vi "ALTS-2015 Authentication Screen.vi"(8 "error in (no error)":errorcluster) -> (0 "error IO":errorcluster, 1 "User Group":T1, 2 "User Name":string, 3 "Valid Login?":bool)   [LabVIEW 2013]
uses:
  Controls/ALTS User Group Enum2.ctl
  Controls/ALTS Poll Control Autentication.ctl
panel:
  out "Time":string
  out "User Group":T1
  in  "Delete":bool
  in  "Edit":bool
  in  "Add":bool
  in  "Cancel":bool
  in  "OK":bool
  in  "Password":string
  in  "User Name":i32(ring) items=["Administrator", "oper", "Ajayvignesh"]
  # "Authentication Screen"
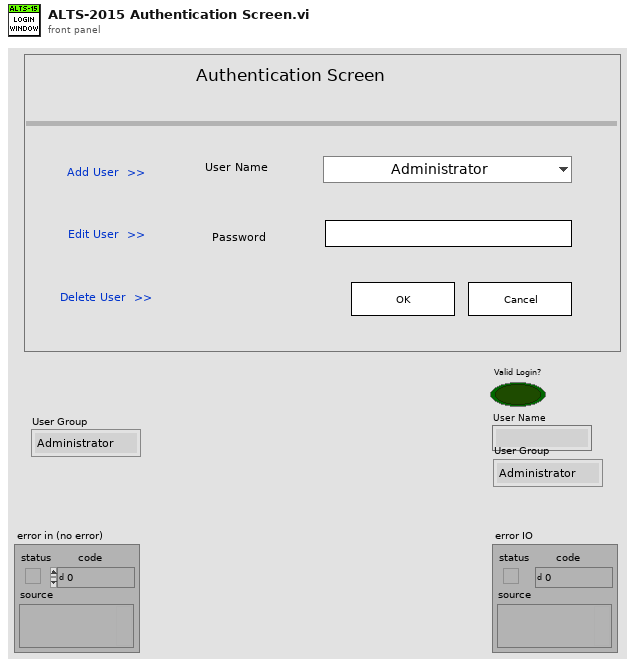
[diagram p1: front panel]
types:
  T1 = typedef "ALTS User Group Enum2.ctl" = enum16{"Administrator", "Super User", "Operator"}
  T2 = typedef "ALTS Poll Control Autentication.ctl" = enum16{">Initialize", ">ReInitialize", ">Poll", ">Handle Error", ">User Name Changed", ">Verify Password", ">On OK", ">On Cancel", ">Add User", ">Edit User", ">Delete User", ">Close Handle", ">NOP", ">Exit"}
  T3 = cluster{"User Names":string, "Password":string, "User Rights":T1}[]
  T4 = typedef "eventvkey.ctl" = enum16{"ASCII", "Enter", "Return", "Shift", "Ctrl", "Alt", "Cmd", "Opt", "Caps", "NumLock", "Clear", "Break", "Up", "Down", "Left", "Right", "Insert", "Delete", "Home", "End", "PageUp", "PageDown", "Escape", "Help", "Pause", "ScrollLock", "F1", "F2", "F3", "F4", "F5", "F6", "F7", "F8", "F9", "F10", "F11", "F12", "F13", "F14", "F15", "F16", "F17", "F18", "F19", "F20", "F21", "F22", "F23", "F24", "Play", "VolumeUp", "VolumeDown", "Mute", "Two Byte Char"}
  T5 = enum16{"OK", "CANCEL", "ABORT", "RETRY", "IGNORE", "YES", "NO"}
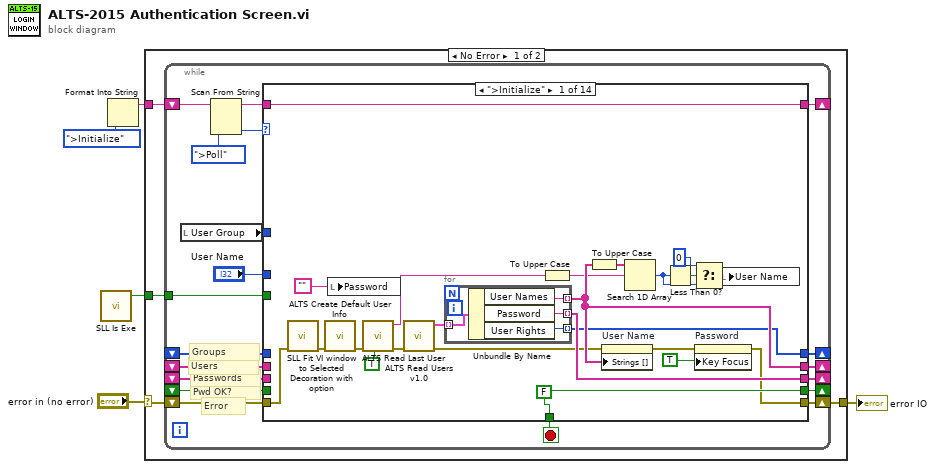
[diagram p0: block diagram]
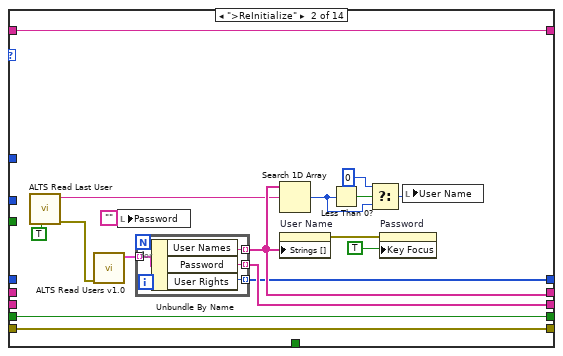
[diagram p2: hidden frame]
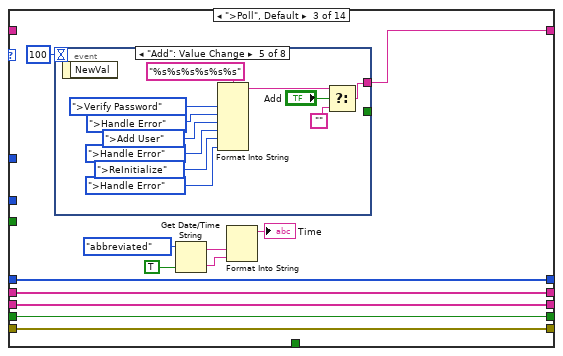
[diagram p3: hidden frame]
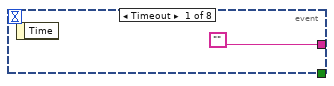
[diagram p4: hidden frame]
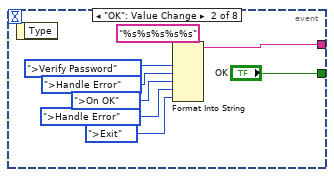
[diagram p5: hidden frame]
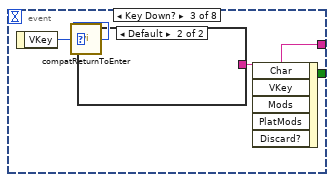
[diagram p6: hidden frame]
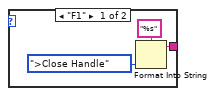
[diagram p7: hidden frame]
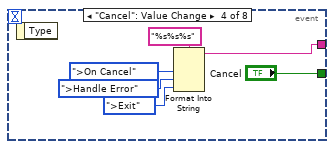
[diagram p8: hidden frame]
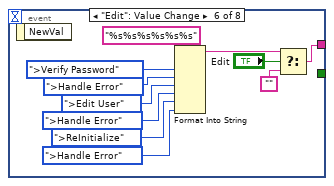
[diagram p9: hidden frame]
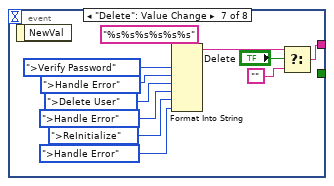
[diagram p10: hidden frame]
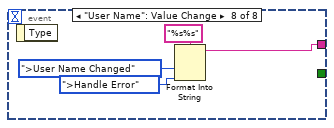
[diagram p11: hidden frame]
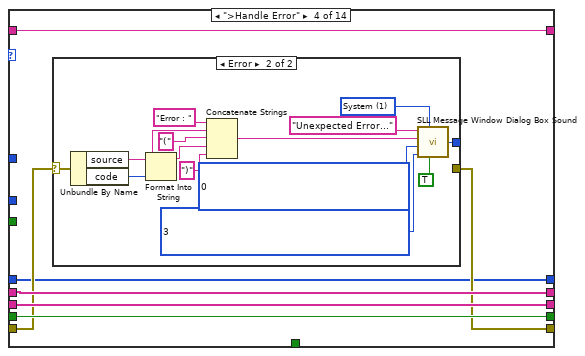
[diagram p12: hidden frame]
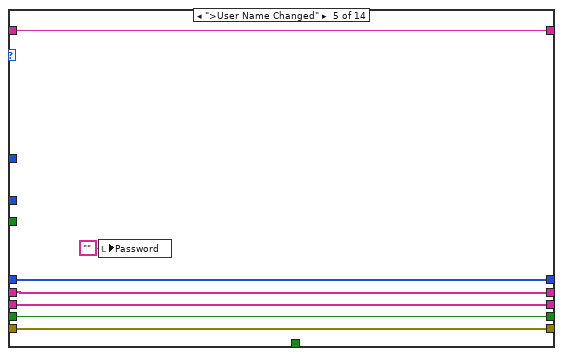
[diagram p14: hidden frame]
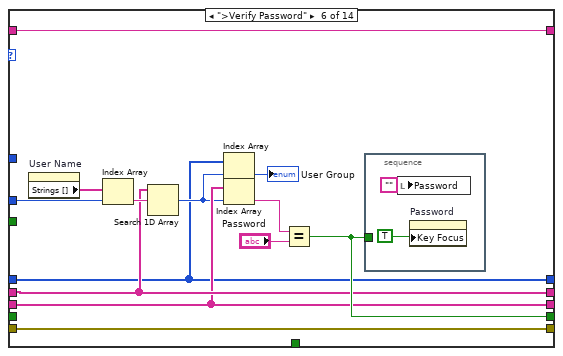
[diagram p15: hidden frame]
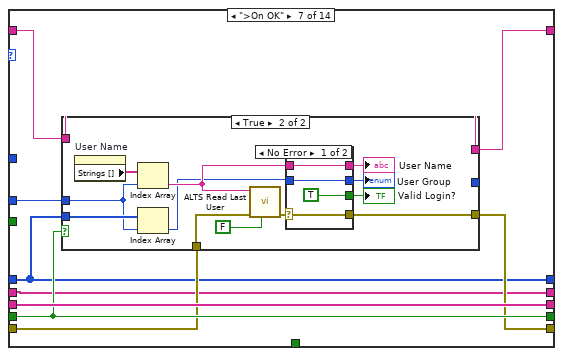
[diagram p16: hidden frame]
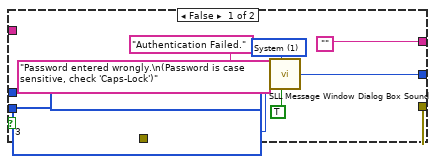
[diagram p17: hidden frame]
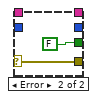
[diagram p18: hidden frame]
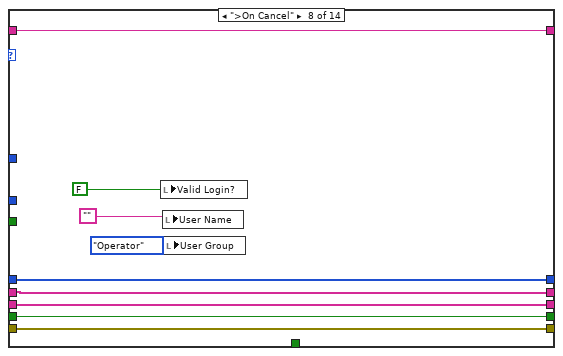
[diagram p19: hidden frame]
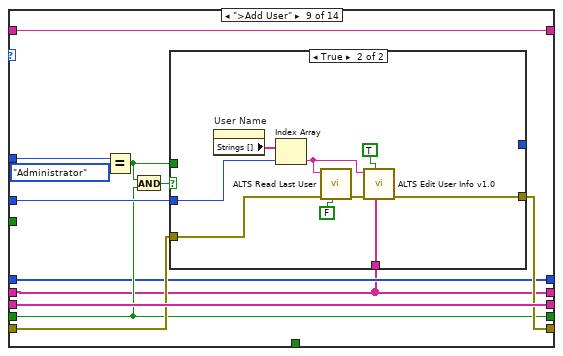
[diagram p20: hidden frame]
diagram:
  n1 = call <userlib>:"SLL Is Exe.vi"() -> ("Is Exe?"=w1:bool)  [unwired: 10 in, 1 out]
  n2 = Format Into String(ALTS_Poll_Control_Autentication.">Initialize" ("Poll Enum Autenticatin")) -> (resulting string=w2:string)  [unwired: 3 in, 1 out]
  n3 = case shown="No Error" "error in (no error)" {
    selector: "error in (no error)" -> [w9 w353]
    tunnel: [w8 w353] -> w4
    tunnel: w2 -> [w7 _]
    tunnel: w1 -> [w6 _]
    frame No Error {
      n4 = while {
        shift-right: [w27] -> w8
        shift-left: w9 -> [w28]
        shift-right: [w22] -> _
        shift-left: w7 -> [w25]
        shift-right: [w16] -> _
        shift-left: _ -> [w15]
        shift-right: [w17] -> _
        shift-left: _ -> [w18]
        shift-right: [w19] -> _
        shift-left: _ -> [w20]
        tunnel: w6 -> [w14]
        shift-right: [w10] -> _
        shift-left: _ -> [w11]
        stop <- w21 stop-if-true
        # "Error"
        # "Pwd OK?"
        # "Passwords"
        # "Users"
        # "Groups"
        n5 = local read "User Group"() -> (w13:T1)
        n6 = Scan From String(input string=w25, default 1=ALTS_Poll_Control_Autentication.">Poll" ("Poll Enum Autenticatin")) -> (remaining string=w23:string, output 1=w24:T2)  [unwired: 3 in, 2 out]
        n7 = case shown="\">Initialize\"" w24 {
          tunnel: [w46 w71 w77 w148 w174 w183 w196 w233 w245 w275 w302 w334 w344 w347] -> w27
          tunnel: w28 -> [w29 w71 w77 w149 w174 w183 w197 w233 w246 w276 w303 w334 w344 w347]
          tunnel: w23 -> [w51 w72 _ w153 w175 w188 w194 w231 w248 w279 w307 w339 w345 w352]
          tunnel: [w51 w72 w78 w153 w175 w188 w193 w231 w248 w279 w307 w339 w345 w352] -> w22
          tunnel: [w49 _ _ _ _ _ _ _ _ _ _ _ _ TRUE] -> w21
          tunnel: w20 -> [_ _ w88 w150 w171 w182 w191 w234 w237 w271 w305 w336 w341 w349]
          tunnel: [w50 w70 w88 w150 w171 w182 w191 w234 w237 w271 w305 w336 w341 w349] -> w19
          tunnel: w18 -> [_ _ w84 w151 w172 w181 w199 w235 w247 w278 w306 w337 w342 w350]
          tunnel: [w48 w69 w84 w151 w172 w181 w199 w235 w247 w278 w306 w337 w342 w350] -> w17
          tunnel: [w49 w67 w87 w152 w173 w185 w198 w236 w242 w277 w304 w338 w343 w351] -> w16
          tunnel: w15 -> [_ w67 w87 w152 w173 _ w198 w236 w242 w277 w304 w338 w343 w351]
          tunnel: w14 -> [_ _ _ _ _ _ _ _ _ _ _ _ _ _]
          tunnel: "User Name" -> [_ _ _ _ _ w184 w195 _ w244 w274 w301 _ _ _]
          tunnel: w13 -> [_ _ _ _ _ _ _ _ w241 w273 w299 _ _ _]
          tunnel: w11 -> [_ _ w85 w147 w169 w179 w192 w232 w238 w272 w300 w335 w340 w348]
          tunnel: [w47 w68 w85 w147 w169 w179 w192 w232 w238 w272 w300 w335 w340 w348] -> w10
          frame ">Initialize" {
            w49 = FALSE
            n8 = call <userlib>:"SLL Fit VI window to Selected Decoration with option.vi"("error in (no error)"=w29) -> ("error out"=w30:errorcluster)  [unwired: 9 in, 1 out]
            n9 = call "ALTS Create Default User Info.vi"("error in"=w30) -> ("error out"=w31:errorcluster)  [unwired: 10 in]
            n10 = local write "Password"("" ("Password")) -> ()
            n11 = call "ALTS Read Last User.vi"("Read?"=TRUE, "error in (no error)"=w31) -> ("error out"=w37:errorcluster, "Last User"=w38:string)  [unwired: 8 in]
            n12 = call "ALTS Read Users v1.0.vi"("error in (no error)"=w37) -> ("error out"=w39:errorcluster, "Users"=w40:T3)  [unwired: 9 in]
            n13 = for {
              tunnel: w40 -> [w55] mode=indexing
              tunnel: [w54] -> w50 mode=indexing
              tunnel: [w53] -> w48 mode=indexing
              tunnel: [w52] -> w47 mode=indexing
              n14 = Unbundle By Name(w55) -> ("User Names"=w54:string, "Password"=w53:string, "User Rights"=w52:T1)
            }
            n15 = To Upper Case(1:w38) -> (0:w41:string)
            n16 = To Upper Case(1:w50) -> (0:w42:string[])
            n17 = property on="User Name" class="Ring (strict)"(error in=w39, "Strings []"=w50) -> (error out=w44:errorcluster)  [unwired: 1 in, 1 out]
            n18 = Search 1D Array(1D array=w42, element=w41) -> (index of element=w33:i32)  [unwired: 1 in]
            n19 = Less Than 0?(x=w33) -> (x < 0?=w35:bool)
            n20 = Select(t=0, s=w35, f=w33) -> (s? t:f=w34:i32)
            n21 = property on="Password" class="Str"(error in=w44, "Key Focus"=TRUE) -> (error out=w46:errorcluster)  [unwired: 1 in, 1 out]
            n22 = local write "User Name"(w34) -> ()
          }
          frame ">ReInitialize" {
            n23 = call "ALTS Read Last User.vi"("Read?"=TRUE) -> ("error out"=w61:errorcluster, "Last User"=w62:string)  [unwired: 9 in]
            n24 = call "ALTS Read Users v1.0.vi"("error in (no error)"=w61) -> ("Users"=w63:T3)  [unwired: 9 in, 1 out]
            n25 = local write "Password"("" ("Password")) -> ()
            n26 = for {
              tunnel: w63 -> [w76] mode=indexing
              tunnel: [w75] -> w70 mode=indexing
              tunnel: [w74] -> w69 mode=indexing
              tunnel: [w73] -> w68 mode=indexing
              n27 = Unbundle By Name(w76) -> ("User Names"=w75:string, "Password"=w74:string, "User Rights"=w73:T1)
            }
            n28 = Search 1D Array(1D array=w70, element=w62) -> (index of element=w58:i32)  [unwired: 1 in]
            n29 = property on="User Name" class="Ring (strict)"("Strings []"=w70) -> (error out=w65:errorcluster)  [unwired: 2 in, 1 out]
            n30 = Less Than 0?(x=w58) -> (x < 0?=w59:bool)
            n31 = Select(t=0, s=w59, f=w58) -> (s? t:f=w56:i32)
            n32 = property on="Password" class="Str"(error in=w65, "Key Focus"=TRUE) -> ()  [unwired: 1 in, 2 out]
            n33 = local write "User Name"(w56) -> ()
          }
          frame ">Poll", Default {
            n34 = event shown="[4] \"Add\": Value Change" {
              selector: _ -> [_ _ _ _ _ _ _ _]
              dyn-events: _ -> [_ _ _ _ _ _ _ _]
              timeout: 100 -> [_ _ _ _ _ _ _ _]
              tunnel: [_ "OK" _ "Cancel" _ _ _ _] -> _
              tunnel: ["" w94 w99 w107 w111 w122 w133 w144] -> w78
              event Timeout {
                n35 = event-data() -> ()  [unwired: 1 in, 1 out]
              }
              event "OK": Value Change {
                n36 = event-data() -> ()  [unwired: 1 in, 1 out]
                n37 = Format Into String(format string="%s%s%s%s%s", ALTS_Poll_Control_Autentication.">Verify Password" ("Poll Enum Autenticatin"), ALTS_Poll_Control_Autentication.">Handle Error" ("Poll Enum Autenticatin"), ALTS_Poll_Control_Autentication.">On OK" ("Poll Enum Autenticatin"), ALTS_Poll_Control_Autentication.">Handle Error" ("Poll Enum Autenticatin"), ALTS_Poll_Control_Autentication.">Exit" ("Poll Enum Autenticatin")) -> (resulting string=w94:string)  [unwired: 2 in, 1 out]
              }
              event Key Down? {
                n38 = event-data() -> ("VKey"=w98:T4)  [unwired: 1 in]
                n39 = call <vilib>:"compatReturnToEnter.vi"("VKey"=w98) -> ("VKey"=w100:T4)
                n40 = case shown="Default" w100 {
                  tunnel: [w101 _] -> w99
                  frame "F1" {
                    n41 = Format Into String(format string="%s", ALTS_Poll_Control_Autentication.">Close Handle" ("Poll Enum Autenticatin")) -> (resulting string=w101:string)  [unwired: 2 in, 1 out]
                  }
                  frame Default {
                  }
                }
                n42 = event-data() -> ()  [unwired: 6 in, 1 out]
              }
              event "Cancel": Value Change {
                n43 = event-data() -> ()  [unwired: 1 in, 1 out]
                n44 = Format Into String(format string="%s%s%s", ALTS_Poll_Control_Autentication.">On Cancel" ("Poll Enum Autenticatin"), ALTS_Poll_Control_Autentication.">Handle Error" ("Poll Enum Autenticatin"), ALTS_Poll_Control_Autentication.">Exit" ("Poll Enum Autenticatin")) -> (resulting string=w107:string)  [unwired: 2 in, 1 out]
              }
              event "Add": Value Change {
                n45 = event-data() -> ()  [unwired: 1 in, 1 out]
                n46 = Format Into String(format string="%s%s%s%s%s%s", ALTS_Poll_Control_Autentication.">Verify Password" ("Poll Enum Autenticatin"), ALTS_Poll_Control_Autentication.">Handle Error" ("Poll Enum Autenticatin"), ALTS_Poll_Control_Autentication.">Add User" ("Poll Enum Autenticatin"), ALTS_Poll_Control_Autentication.">Handle Error" ("Poll Enum Autenticatin"), ALTS_Poll_Control_Autentication.">ReInitialize" ("Poll Enum Autenticatin"), ALTS_Poll_Control_Autentication.">Handle Error" ("Poll Enum Autenticatin")) -> (resulting string=w113:string)  [unwired: 2 in, 1 out]
                n47 = Select(t=w113, s="Add", f="") -> (s? t:f=w111:string)
              }
              event "Edit": Value Change {
                n48 = event-data() -> ()  [unwired: 1 in, 1 out]
                n49 = Format Into String(format string="%s%s%s%s%s%s", ALTS_Poll_Control_Autentication.">Verify Password" ("Poll Enum Autenticatin"), ALTS_Poll_Control_Autentication.">Handle Error" ("Poll Enum Autenticatin"), ALTS_Poll_Control_Autentication.">Edit User" ("Poll Enum Autenticatin"), ALTS_Poll_Control_Autentication.">Handle Error" ("Poll Enum Autenticatin"), ALTS_Poll_Control_Autentication.">ReInitialize" ("Poll Enum Autenticatin"), ALTS_Poll_Control_Autentication.">Handle Error" ("Poll Enum Autenticatin")) -> (resulting string=w124:string)  [unwired: 2 in, 1 out]
                n50 = Select(t=w124, s="Edit", f="") -> (s? t:f=w122:string)
              }
              event "Delete": Value Change {
                n51 = event-data() -> ()  [unwired: 1 in, 1 out]
                n52 = Format Into String(format string="%s%s%s%s%s%s", ALTS_Poll_Control_Autentication.">Verify Password" ("Poll Enum Autenticatin"), ALTS_Poll_Control_Autentication.">Handle Error" ("Poll Enum Autenticatin"), ALTS_Poll_Control_Autentication.">Delete User" ("Poll Enum Autenticatin"), ALTS_Poll_Control_Autentication.">Handle Error" ("Poll Enum Autenticatin"), ALTS_Poll_Control_Autentication.">ReInitialize" ("Poll Enum Autenticatin"), ALTS_Poll_Control_Autentication.">Handle Error" ("Poll Enum Autenticatin")) -> (resulting string=w135:string)  [unwired: 2 in, 1 out]
                n53 = Select(t=w135, s="Delete", f="") -> (s? t:f=w133:string)
              }
              event "User Name": Value Change {
                n54 = event-data() -> ()  [unwired: 1 in, 1 out]
                n55 = Format Into String(format string="%s%s", ALTS_Poll_Control_Autentication.">User Name Changed" ("Poll Enum Autenticatin"), ALTS_Poll_Control_Autentication.">Handle Error" ("Poll Enum Autenticatin")) -> (resulting string=w144:string)  [unwired: 2 in, 1 out]
              }
            }
            n56 = Get Date/Time String(date format (0)=enum16{"short", "long", "abbreviated"}."abbreviated", want seconds? (F)=TRUE) -> (date string=w82:string, time string=w81:string)  [unwired: 1 in]
            n57 = Format Into String(w82, w81) -> (resulting string=→"Time":string)  [unwired: 3 in, 1 out]
          }
          frame ">Handle Error" {
            n58 = case shown="Error" w149 {
              selector: w149 -> [w154 w163]
              tunnel: [w154 _] -> w148
              tunnel: [_ w155] -> _
              frame No Error {
              }
              frame Error {
                w165 = 1 items=["Application", "System", "Task"] ("modality (0)")
                n59 = Unbundle By Name(w163) -> ("source"=w161:string, "code"=w162:i32)
                n60 = Format Into String(w162) -> (resulting string=w160:string)  [unwired: 3 in, 1 out]
                n61 = Concatenate Strings("Error : " ("string"), w161, "(" ("string"), w160, ")" ("string")) -> (w156:string)
                n62 = call <userlib>:"SLL Message Window Dialog Box Sound.vi"("Sound? (F)"=TRUE ("sound? (F)"), "Modality (0)"=w165, "Icon (0:None)"=3 ("icon (0:None)"), "Buttons (0:OK)"=0 ("buttons (0:OK)"), "Message (\"\")"=w156, "Window Title (\"\")"="Unexpected Error..." ("window title (\"\")")) -> ("Button Pressed"=w155:T5)
              }
            }
          }
          frame ">User Name Changed" {
            n63 = local write "Password"("") -> ()
          }
          frame ">Verify Password" {
            n64 = property on="User Name" class="Ring (strict)"() -> ("Strings []"=w186:string[])  [unwired: 2 in, 2 out]
            n65 = Index Array(array=w186, index=w184) -> (element=w187:string)
            n66 = Search 1D Array(1D array=w182, element=w187) -> (index of element=w180:i32)  [unwired: 1 in]
            n67 = Index Array(array=w179, index=w180) -> (element=→"User Group":T1)
            n68 = Index Array(array=w181, index=w180) -> (element=w177:string)
            n69 = Equal?(x=w177, y="Password") -> (x = y?=w185:bool)
            n70 = stacked-sequence {
              tunnel: w185 -> [_]
              frame #0 {
                n71 = local write "Password"("" ("Password")) -> ()
                n72 = property on="Password" class="Str"("Key Focus"=TRUE) -> ()  [unwired: 2 in, 2 out]
              }
            }
          }
          frame ">On OK" {
            n73 = case shown="True" w198 {
              tunnel: [w208 _] -> _
              tunnel: w197 -> [w201 w219]
              tunnel: [w201 w213] -> w196
              tunnel: w195 -> [_ w214]
              tunnel: ["" w218] -> w193
              tunnel: w194 -> [_ w218]
              tunnel: w192 -> [_ w216]
              frame False {
                w203 = 1 items=["Application", "System", "Task"] ("modality (0)")
                n74 = call <userlib>:"SLL Message Window Dialog Box Sound.vi"("Sound? (F)"=TRUE ("sound? (F)"), "Modality (0)"=w203, "Icon (0:None)"=3 ("icon (0:None)"), "Buttons (0:OK)"=0 ("buttons (0:OK)"), "Message (\"\")"="Password entered wrongly.\n(Password is case sensitive, check 'Caps-Lock')" ("message (\"\")"), "Window Title (\"\")"="Authentication Failed." ("window title (\"\")")) -> ("Button Pressed"=w208:T5)
              }
              frame True {
                n75 = property on="User Name" class="Ring (strict)"() -> ("Strings []"=w221:string[])  [unwired: 2 in, 2 out]
                n76 = Index Array(array=w221, index=w214) -> (element=w217:string)
                n77 = Index Array(array=w216, index=w214) -> (element=w210:T1)
                n78 = call "ALTS Read Last User.vi"("Read?"=FALSE, "error in (no error)"=w219, "Last User"=w217) -> ("error out"=w215:errorcluster)  [unwired: 7 in, 1 out]
                n79 = case shown="No Error" w215 {
                  selector: w215 -> [w225 w226]
                  tunnel: w217 -> [w223 _]
                  tunnel: w210 -> [w222 _]
                  tunnel: [w225 w226] -> w213
                  tunnel: [TRUE ("Valid Login?") FALSE ("Valid Login?")] -> w209
                  tunnel: [w223 _] -> w212
                  tunnel: [w222 _] -> w211
                  frame No Error {
                  }
                  frame Error {
                  }
                }
                "User Name" <- w212
                "User Group" <- w211
                "Valid Login?" <- w209
              }
            }
          }
          frame ">On Cancel" {
            n80 = local write "Valid Login?"(FALSE ("Valid Login?")) -> ()
            n81 = local write "User Name"("") -> ()
            n82 = local write "User Group"(ALTS_User_Group_Enum2."Operator" ("User Group")) -> ()
          }
          frame ">Add User" {
            n83 = Equal?(x=w241, y=ALTS_User_Group_Enum2."Administrator" ("User Group")) -> (x = y?=w239:bool)
            n84 = And(x=w239, y=w242) -> (x .and. y?=w243:bool)
            n85 = case shown="True" w243 {
              tunnel: [w257 _] -> _
              tunnel: w246 -> [w250 w267]
              tunnel: [w250 w270] -> w245
              tunnel: w244 -> [_ w269]
              tunnel: w239 -> [w249 _]
              tunnel: w237 -> [_ w268]
              frame False {
                w252 = 1 items=["Application", "System", "Task"] ("modality (0)")
                n86 = case shown="False" w249 {
                  tunnel: ["Password entered wrongly.\nYou must authenticate to edit user information." ("message (\"\")") " You don't have sufficient rights for this operation." ("message (\"\")")] -> w254
                  tunnel: ["Authentication Failed..." ("window title (\"\")") "Access Denied" ("window title (\"\")")] -> w253
                  frame True {
                  }
                  frame False {
                  }
                }
                n87 = call <userlib>:"SLL Message Window Dialog Box Sound.vi"("Sound? (F)"=TRUE ("sound? (F)"), "Modality (0)"=w252, "Icon (0:None)"=3 ("icon (0:None)"), "Buttons (0:OK)"=0 ("buttons (0:OK)"), "Message (\"\")"=w254, "Window Title (\"\")"=w253) -> ("Button Pressed"=w257:T5)
              }
              frame True {
                n88 = property on="User Name" class="Ring (strict)"() -> ("Strings []"=w265:string[])  [unwired: 2 in, 2 out]
                n89 = Index Array(array=w265, index=w269) -> (element=w264:string)
                n90 = call "ALTS Read Last User.vi"("Read?"=FALSE, "error in (no error)"=w267, "Last User"=w264) -> ("error out"=w263:errorcluster)  [unwired: 7 in, 1 out]
                n91 = call "ALTS Edit User Info v1.0.vi"("Users"=w268, "Add(T)/Edit(F)"=TRUE, "error in (no error)"=w263, "User Name"=w264) -> ("error out"=w270:errorcluster)  [unwired: 7 in]
              }
            }
          }
          frame ">Edit User" {
            n92 = case shown="True" w277 {
              tunnel: [w287 _] -> _
              tunnel: w276 -> [w280 w289]
              tunnel: [w280 w298] -> w275
              tunnel: w274 -> [_ w297]
              tunnel: w273 -> [_ w296]
              tunnel: w271 -> [_ w295]
              frame False {
                w282 = 1 items=["Application", "System", "Task"] ("modality (0)")
                n93 = call <userlib>:"SLL Message Window Dialog Box Sound.vi"("Sound? (F)"=TRUE ("sound? (F)"), "Modality (0)"=w282, "Icon (0:None)"=3 ("icon (0:None)"), "Buttons (0:OK)"=0 ("buttons (0:OK)"), "Message (\"\")"="Password entered wrongly.\nYou must authenticate to edit user information." ("message (\"\")"), "Window Title (\"\")"="Authentication Failed..." ("window title (\"\")")) -> ("Button Pressed"=w287:T5)
              }
              frame True {
                n94 = property on="User Name" class="Ring (strict)"() -> ("Strings []"=w293:string[])  [unwired: 2 in, 2 out]
                n95 = Index Array(array=w293, index=w297) -> (element=w292:string)
                n96 = call "ALTS Read Last User.vi"("Read?"=FALSE, "error in (no error)"=w289, "Last User"=w292) -> ("error out"=w288:errorcluster, "Last User"=w291:string)  [unwired: 7 in]
                n97 = call "ALTS Edit User Info v1.0.vi"("Users"=w295, "Add(T)/Edit(F)"=FALSE, "error in (no error)"=w288, "User Group"=w296, "User Name"=w291) -> ("error out"=w298:errorcluster)  [unwired: 6 in]
              }
            }
          }
          frame ">Delete User" {
            n98 = case shown="True" w304 {
              tunnel: [w315 _] -> _
              tunnel: w303 -> [w308 w321]
              tunnel: [w308 w320] -> w302
              tunnel: w301 -> [_ w317]
              tunnel: w299 -> [_ w319]
              frame False {
                w310 = 1 items=["Application", "System", "Task"] ("modality (0)")
                n99 = call <userlib>:"SLL Message Window Dialog Box Sound.vi"("Sound? (F)"=TRUE ("sound? (F)"), "Modality (0)"=w310, "Icon (0:None)"=3 ("icon (0:None)"), "Buttons (0:OK)"=0 ("buttons (0:OK)"), "Message (\"\")"="Password entered wrongly.\nYou must authenticate to edit user information." ("message (\"\")"), "Window Title (\"\")"="Authentication Failed..." ("window title (\"\")")) -> ("Button Pressed"=w315:T5)
              }
              frame True {
                n100 = property on="User Name" class="Ring (strict)"() -> ("Strings []"=w318:string[])  [unwired: 2 in, 2 out]
                n101 = Index Array(array=w318, index=w317) -> (element=w316:string)
                n102 = case shown="\"Operator\", Default" w319 {
                  tunnel: w321 -> [w325 w333]
                  tunnel: [w326 w333] -> w320
                  tunnel: [_ w332] -> _
                  tunnel: w316 -> [w322 _]
                  frame "Administrator" {
                    n103 = call "ALTS Read Last User.vi"("Read?"=FALSE, "error in (no error)"=w325, "Last User"=w322) -> ("error out"=w323:errorcluster)  [unwired: 7 in, 1 out]
                    n104 = call "ALTS Delete User Account v1.0.vi"("error in (no error)"=w323, "Last User"=w322) -> ("error out"=w326:errorcluster)  [unwired: 9 in]
                  }
                  frame "Operator", Default {
                    w330 = 1 items=["Application", "System", "Task"] ("modality (0)")
                    n105 = call <userlib>:"SLL Message Window Dialog Box Sound.vi"("Modality (0)"=w330, "Icon (0:None)"=3 ("icon (0:None)"), "Buttons (0:OK)"=0 ("buttons (0:OK)"), "Message (\"\")"=" You don't have sufficient rights for this operation." ("message (\"\")"), "Window Title (\"\")"="Acess Denied." ("window title (\"\")")) -> ("Button Pressed"=w332:T5)  [unwired: 1 in]
                  }
                }
              }
            }
          }
          frame ">Close Handle" {
          }
          frame ">NOP" {
          }
          frame ">Exit" {
          }
        }
      }
    }
    frame Error {
    }
  }
  "error IO" <- w4
